vi "GetClientServerTemplateBuildSpecPath.vi"(11 "Base Path":path) -> (3 "ClientServerTemplateBuildSpecPath":path)   [LabVIEW 2019]
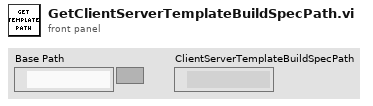
[diagram p1: front panel]
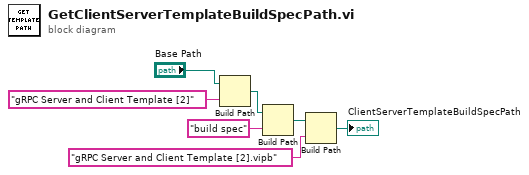
[diagram p0: block diagram]
diagram:
  n1 = Build Path(base path="Base Path", name or relative path="gRPC Server and Client Template [2]") -> (appended path=w3:path)
  n2 = Build Path(base path=w3, name or relative path="build spec") -> (appended path=w5:path)
  n3 = Build Path(base path=w5, name or relative path="gRPC Server and Client Template [2].vipb") -> (appended path=→"ClientServerTemplateBuildSpecPath":path)
